vi "Live window-Cleanup.vi"(10 "Stop":bool, 11 "Boolean":bool) -> (0 "error out":errorcluster)   [LabVIEW 2013]
uses:
  Global Variables/General Globals.vi
  Globals/gl_Windows Ctrl refs.vi
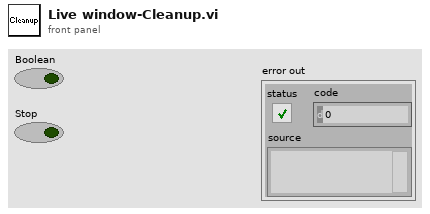
[diagram p1: front panel]
types:
  T1 = typedef "Live window-ctrl refs.ctl" = cluster{"This VI":refnum<vi>, "Pane":refnum<vi>, "Snapshot":refnum<vi>, "Left Image Palette":refnum<vi>, "Right Image Palette":refnum<vi>, "Left Channel":refnum<vi>, "Right Channel":refnum<vi>, "Left image intensity":refnum<vi>, "Right image intensity":refnum<vi>, "Left Image Display":T2, "Right Image Display":T2, "Refresh rate ind (Hz)":refnum<vi>, "Acq rate ind (Hz)":refnum<vi>, "Stop (ind)":refnum<vi>}
  T2 = typedef "Image display ref.ctl" = refnum<vi>
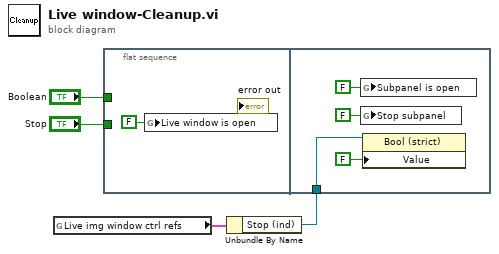
[diagram p0: block diagram]
diagram:
  n1 = global read "gl_Windows Ctrl refs.vi" "Live img window ctrl refs"() -> (w2:T1)
  n2 = flat-sequence {
    tunnel: "Boolean" -> [_]
    tunnel: "Stop" -> [_]
    tunnel: w1 -> [w6]
    frame #0 {
      n3 = global write "General Globals.vi" "Live window is open"(FALSE ("Live window running")) -> ()
    }
    frame #1 {
      n4 = global write "General Globals.vi" "Subpanel is open"(FALSE ("Subpanel is open")) -> ()
      n5 = global write "General Globals.vi" "Stop subpanel"(FALSE ("Stop subpanel")) -> ()
      n6 = property class="Bool (strict)"(reference=w6, "Value"=FALSE ("Stop (ind)")) -> ()  [unwired: 1 in, 2 out]
    }
  }
  n7 = Unbundle By Name(w2) -> ("Stop (ind)"=w1:refnum<vi>)
